vi "Get_array_values_fr_String.vi"(0 "String Value":string) -> (1 "Numeric Array":dbl[](array[numeric]) format="%.2f", 2 "String array":string[](array[string]))   [LabVIEW 2010]
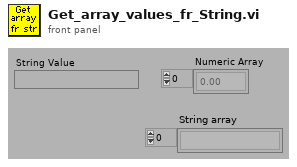
[diagram p1: front panel]
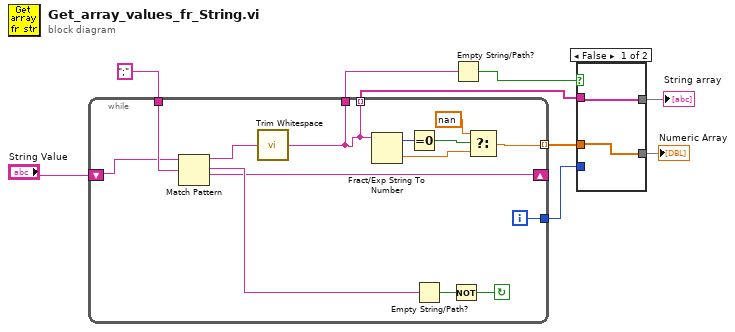
[diagram p0: block diagram]
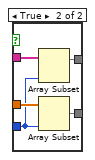
[diagram p2: hidden frame]
diagram:
  n1 = while {
    tunnel: [w10] -> w2
    tunnel: [w11] -> w5
    tunnel: [w10] -> w3 mode=indexing
    tunnel: [w13] -> w7 mode=indexing
    shift-left: "String Value" -> [w19]
    shift-right: [w18] -> _
    tunnel: ";" ("regular expression") -> [w23]
    i -> [w11]
    stop <- w20 continue-if-true
    n2 = Match Pattern(string=w19, regular expression=w23) -> (before substring=w17:string, match substring=w22:string, after substring=w18:string)  [unwired: 2 out]
    n3 = call <vilib>:"Trim Whitespace.vi"("string"=w17) -> ("trimmed string"=w10:string)  [unwired: 1 in]
    n4 = Fract/Exp String To Number(string=w10) -> (offset past number=w16:i32, number=w14:dbl)  [unwired: 1 in, 2 out]
    n5 = Equal To 0?(x=w16) -> (x = 0?=w15:bool)
    n6 = Empty String/Path?(string/path=w22) -> (empty?=w21:bool)
    n7 = Not(x=w21) -> (.not. x?=w20:bool)
    n8 = Select(t=nan, s=w15, f=w14) -> (s? t:f=w13:dbl)
  }
  n9 = Empty String/Path?(string/path=w2) -> (empty?=w1:bool)
  n10 = case shown="False" w1 {
    tunnel: w7 -> [w24 w30]
    tunnel: [w24 w29] -> w6
    tunnel: w5 -> [_ w28]
    tunnel: [w25 w27] -> w4
    tunnel: w3 -> [w25 w26]
    frame False {
    }
    frame True {
      n11 = Array Subset(array=w26, length=w28) -> (w27:string[])  [unwired: 1 in]
      n12 = Array Subset(array=w30, length=w28) -> (w29:dbl[])  [unwired: 1 in]
    }
  }
  "Numeric Array" <- w6
  "String array" <- w4
